vi "FCI_Cam_1_Coordinate_System.vi"(0 "ROI":T1, 5 "Edge Options":T5={"Edge Polarity"=2, "Kernel Size"=3, "Width"=3, "Minimum Edge Strength"=50.0, "Interpolation Type"=enum."Zero Order", "Data Processing Method"=enum."Average"} {"Edge Polarity" items=["All Edges", "Rising Edges", "Falling Edges"]; "Minimum Edge Strength" format="%.2f"; "Width" step=2; "Kernel Size" step=2}, 7 "Line Options":T3={"Number of Lines"=1, "Type"=enum."Best Edge Rake", "Min. Score"=10.0, "Max. Score"=1000.0, "Orientation"=0.0, "Angle Range"=60.0, "Angle Tolerance"=1.0, "Step Size"=18, "Min. SNR (db)"=0.0, "Min. Points (%)"=25.0, "Hough Iterations"=5} {"Min. Points (%)" min=0.0 max=100.0; "Min. SNR (db)" min=0.0; "Max. Score" min=0.0 max=1024.0; "Min. Score" min=0.0 max=1024.0 step=1.0}, 9 "Search Direction":u32(ring)=2 items=["Left to Right", "Right to Left", "Top to Bottom", "Bottom to Top"], 11 "error in (no error)":errorcluster) -> (4 "Coordinate System":T2 {"Axis Reference" items=["Direct", "Indirect"]; "Angle (deg)" format="%.2f"; "Origin"."Y" format="%.2f"; "Origin"."X" format="%.2f"}, 15 "error out":errorcluster)   [LabVIEW 2015]
uses:
  <vilib>/vision/Measure.llb/Edge Options.ctl
  <vilib>/vision/Measure.llb/Edge Polarity.ctl
  <vilib>/vision/Measure.llb/Straight Edge Options.ctl
  <vilib>/vision/Measure.llb/Straight Edge Process.ctl
  <vilib>/vision/NI_Vision_Development_Module.lvlib
  FrameworkOverrides/Algorithm.lvclass
panel:
  in  "Image Out":T7(plugin-control)
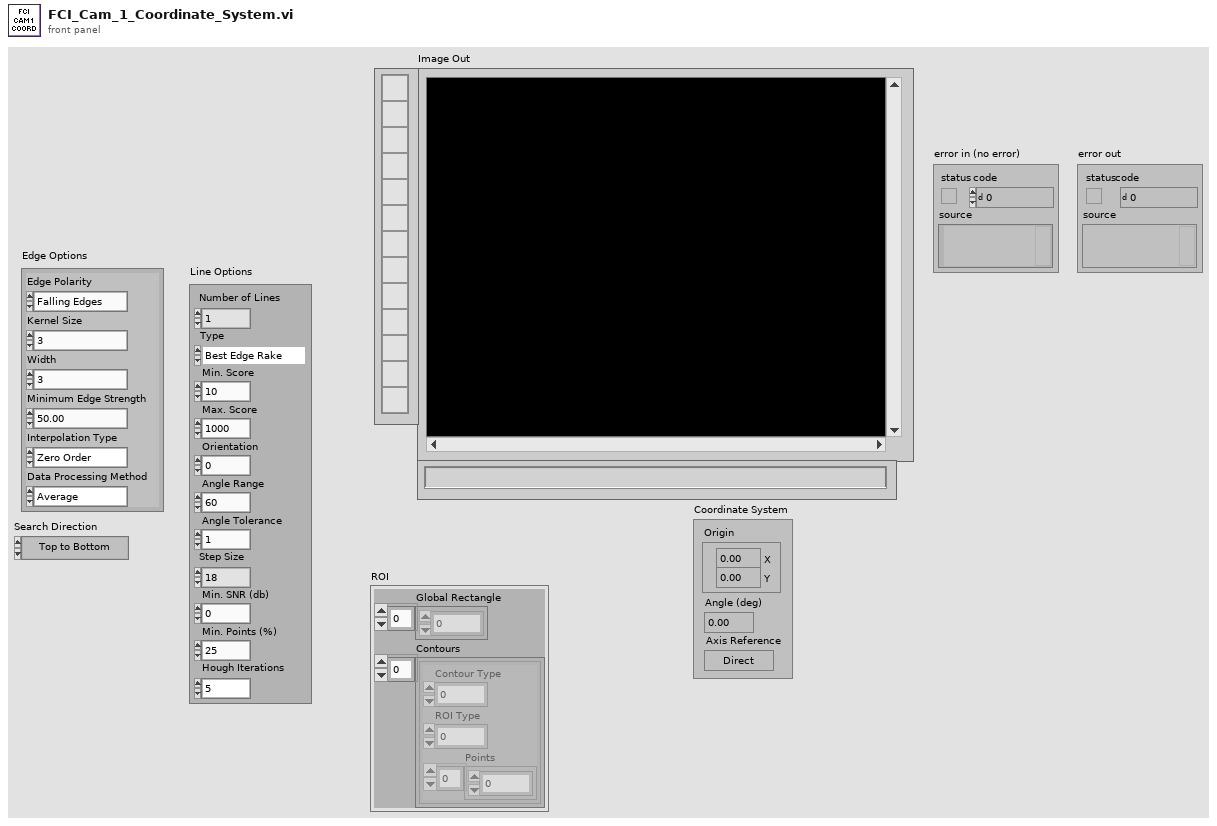
[diagram p1: front panel]
types:
  T1 = cluster{"Global Rectangle":i32[], "Contours":cluster{"Contour Type":u32, "ROI Type":u32, "Points":i32[]}[]}
  T2 = cluster{"Origin":cluster{"X":sgl, "Y":sgl}, "Angle (deg)":sgl, "Axis Reference":u32}
  T3 = typedef "Straight Edge Options.ctl" = cluster{"Number of Lines":i32, "Type":T4, "Min. Score":dbl, "Max. Score":dbl, "Orientation":dbl, "Angle Range":dbl, "Angle Tolerance":dbl, "Step Size":u32, "Min. SNR (db)":dbl, "Min. Points (%)":dbl, "Hough Iterations":i32}
  T4 = typedef "Straight Edge Process.ctl" = enum32{"First Edge Rake", "Best Edge Rake", "Hough Edge Rake", "First Edge Projection", "Best Edge Projection"}
  T5 = typedef "Edge Options.ctl" = cluster{"Edge Polarity":T6, "Kernel Size":u32, "Width":u32, "Minimum Edge Strength":sgl, "Interpolation Type":enum32{"Zero Order", "Bilinear", "Quadratic", "Cubic", "Bilinear Fixed"}, "Data Processing Method":enum32{"Average", "Median"}}
  T6 = typedef "Edge Polarity.ctl" = u32
  T7 = typedef "IMAQ Image.ctl" = refnum<image>
  T8 = cluster{"Point1 (Pixels)":cluster{"X":sgl, "Y":sgl}, "Point2 (Pixels)":cluster{"X":sgl, "Y":sgl}, "Point1 (Real-World)":cluster{"X":sgl, "Y":sgl}, "Point2 (Real-World)":cluster{"X":sgl, "Y":sgl}, "Angle (Pixel)":dbl, "Angle (Real-World)":dbl, "Score":dbl, "Straightness":dbl, "Average SNR (db)":dbl, "Calibration Valid":bool}[]
  T9 = cluster{"Point1 (Pixels)":cluster{"X":sgl, "Y":sgl}, "Point2 (Pixels)":cluster{"X":sgl, "Y":sgl}, "Point1 (Real-World)":cluster{"X":sgl, "Y":sgl}, "Point2 (Real-World)":cluster{"X":sgl, "Y":sgl}, "Angle (Pixel)":dbl, "Angle (Real-World)":dbl, "Score":dbl, "Straightness":dbl, "Average SNR (db)":dbl, "Calibration Valid":bool}
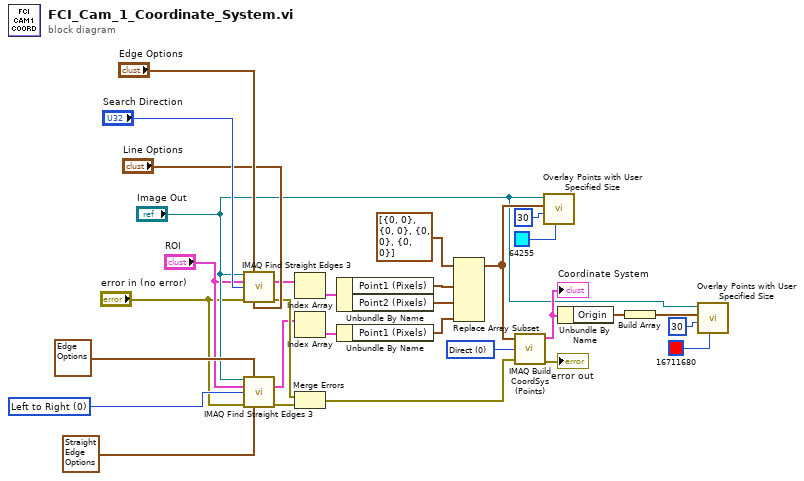
[diagram p0: block diagram]
diagram:
  w27 = u32 0 items=["Left to Right", "Right to Left", "Top to Bottom", "Bottom to Top"] ("Search Direction 2")
  w17 = u32 0 items=["Direct", "Indirect"] ("Axis Reference")
  n1 = call "IMAQ Find Straight Edges 3"("Image"="Image Out", "Edge Options"="Edge Options", "ROI Descriptor"="ROI", "Search Direction"="Search Direction", "error in (no error)"="error in (no error)", "Line Options"="Line Options") -> ("Straight Edges"=w21:T8, "error out"=w24:errorcluster)  [unwired: 5 in, 3 out]
  n2 = call "IMAQ Find Straight Edges 3"("Image"="Image Out", "Edge Options"=T5 {"Edge Polarity"=2, "Kernel Size"=3, "Width"=3, "Minimum Edge Strength"=50.0, "Interpolation Type"=enum."Zero Order", "Data Processing Method"=enum."Average"} ("Edge Options 2"), "ROI Descriptor"="ROI", "Search Direction"=w27, "error in (no error)"="error in (no error)", "Line Options"=T3 {"Number of Lines"=1, "Type"=enum."First Edge Rake", "Min. Score"=10.0, "Max. Score"=1000.0, "Orientation"=0.0, "Angle Range"=70.0, "Angle Tolerance"=1.0, "Step Size"=15, "Min. SNR (db)"=0.0, "Min. Points (%)"=25.0, "Hough Iterations"=5} ("Line Options 2")) -> ("Straight Edges"=w19:T8, "error out"=w23:errorcluster)  [unwired: 5 in, 3 out]
  n3 = Index Array(array=w21) -> (element=w20:T9)  [unwired: 1 in]
  n4 = Index Array(array=w19) -> (element=w18:T9)  [unwired: 1 in]
  n5 = Merge Errors(w24, w23) -> (w3:errorcluster)
  n6 = Unbundle By Name(w20) -> ("Point1 (Pixels)"=w6:cluster{"X":sgl, "Y":sgl}, "Point2 (Pixels)"=w5:cluster{"X":sgl, "Y":sgl})
  n7 = Unbundle By Name(w18) -> ("Point1 (Pixels)"=w4:cluster{"X":sgl, "Y":sgl})
  n8 = Replace Array Subset(array=cluster{"X":i32, "Y":i32}[] [{"X"=0, "Y"=0}, {"X"=0, "Y"=0}, {"X"=0, "Y"=0}, {"X"=0, "Y"=0}] ("Reference Points"), new element #1=w6, new element #2=w5, new element #3=w4) -> (w8:cluster{"X":i32, "Y":i32}[])  [unwired: 3 in]
  n9 = call "IMAQ Build CoordSys (Points)"("Reference Points"=w8, "Axis Reference"=w17, "error in (no error)"=w3) -> ("Coordinate System"=w15:T2, "error out"=→"error out":errorcluster)  [unwired: 2 in]
  "Coordinate System" <- w15
  n10 = call "Overlay Points with User Specified Size.vi"("Color"=u32 64255, "Point Diameter (5)"=u32 30, "Points"=w8, "Image In"="Image Out") -> ()  [unwired: 6 in, 2 out]
  n11 = Unbundle By Name(w15) -> ("Origin"=w14:cluster{"X":sgl, "Y":sgl})
  n12 = Build Array(w14) -> (w13:cluster{"X":sgl, "Y":sgl}[])
  n13 = call "Overlay Points with User Specified Size.vi"("Color"=u32 16711680, "Point Diameter (5)"=u32 30, "Points"=w13, "Image In"="Image Out") -> ()  [unwired: 6 in, 2 out]
